vi "fgv_binary-sum-gap_out.vi"(7 "cmd":enum16{"read", "write"}(ring), 11 "binary sum gap":i64) -> (3 "binary sum gap out":i64)   [LabVIEW 2019]
panel:
  out "웨이브폼 차트":i64(graph)
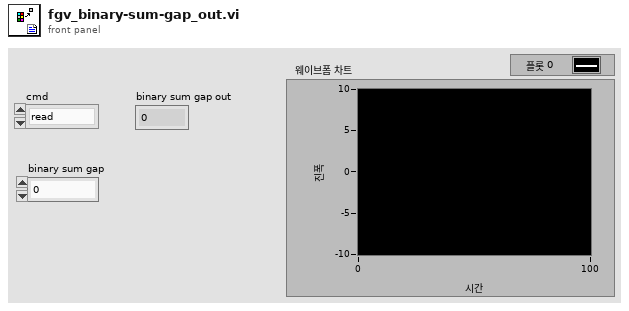
[diagram p1: front panel]
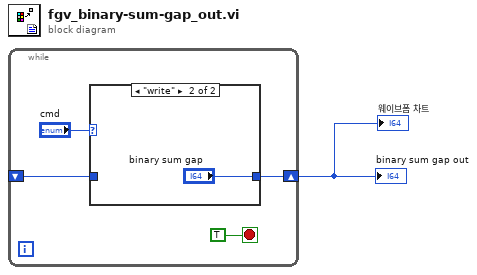
[diagram p0: block diagram]
diagram:
  n1 = while {
    shift-right: [w3] -> w1
    shift-left: _ -> [w2]
    stop <- TRUE stop-if-true
    n2 = case shown="\"write\"" "cmd" {
      tunnel: [w6 "binary sum gap"] -> w3
      tunnel: w2 -> [w6 _]
      frame "read", Default {
      }
      frame "write" {
      }
    }
  }
  "binary sum gap out" <- w1
  "웨이브폼 차트" <- w1
